vi "CheckForValidPath.vi"(0 "Input VI Path":path, 11 "Error In":errorcluster) -> (4 "Front Panel Reference":refnum<vi>, 6 "VI Reference Out":refnum<vi>, 15 "Error Out":errorcluster)   [LabVIEW 2019, in "JsonToCluster.lvlib"]
doc: "This VI returns the front panel reference of a specified VI if the provided path is valid. If the path is invalid or the VI doesn't exist, it creates a new VI and returns its front panel reference."
uses:
  JsonToCluster.lvlib
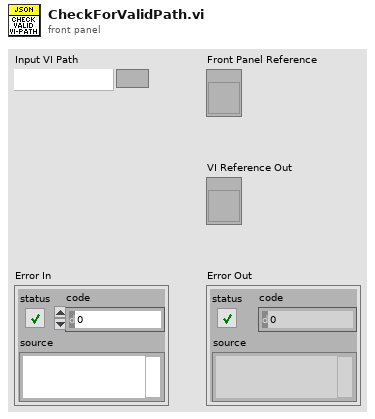
[diagram p1: front panel]
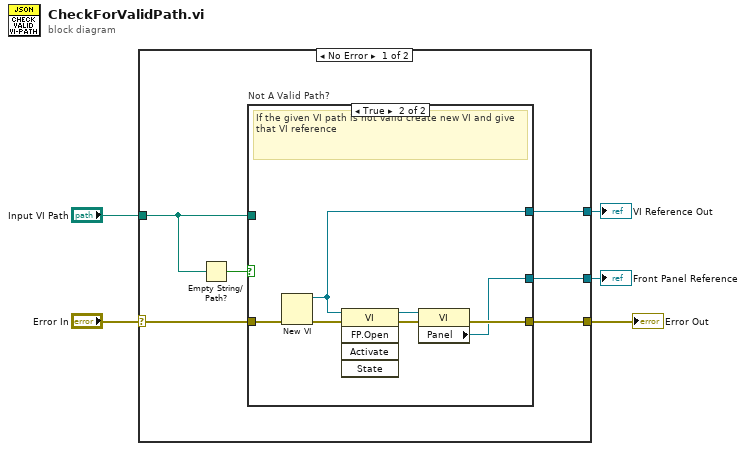
[diagram p0: block diagram]
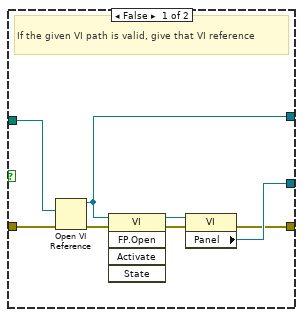
[diagram p2: hidden frame]
diagram:
  n1 = case shown="No Error" "Error In" {
    selector: "Error In" -> [w11 w27]
    tunnel: "Input VI Path" -> [w8 _]
    tunnel: [w10 w27] -> w3
    tunnel: [w9 _] -> w2
    tunnel: [w6 _] -> w1
    frame No Error {
      n2 = Empty String/Path?(string/path=w8) -> (empty?=w7:bool)
      n3 = case "Not A Valid Path?" shown="True" w7 {
        tunnel: w11 -> [w19 w26]
        tunnel: w8 -> [w18 _]
        tunnel: [w14 w21] -> w9
        tunnel: [w13 w22] -> w10
        tunnel: [w12 w20] -> w6
        frame False {
          # "If the given VI path is valid, give that VI reference"
          n4 = Open VI Reference(vi path=w18, error in (no error)=w19) -> (vi reference=w12:refnum<vi>, error out=w15:errorcluster)  [unwired: 4 in]
          n5 = invoke class="VI" method="FP.Open"(reference=w12, error in=w15) -> (reference out=w16:refnum<vi>, error out=w17:errorcluster)  [unwired: 3 in, 3 out]
          n6 = property class="VI"(reference=w16, error in=w17) -> (error out=w13:errorcluster, "Panel"=w14:refnum<vi>)  [unwired: 1 out]
        }
        frame True {
          # "If the given VI path is not valid create new VI and give that VI reference"
          n7 = New VI(8:w26) -> (0:w25:errorcluster, 3:w20:refnum<vi>)  [unwired: 6 in]
          n8 = invoke class="VI" method="FP.Open"(reference=w20, error in=w25) -> (reference out=w23:refnum<vi>, error out=w24:errorcluster)  [unwired: 3 in, 3 out]
          n9 = property class="VI"(reference=w23, error in=w24) -> (error out=w22:errorcluster, "Panel"=w21:refnum<vi>)  [unwired: 1 out]
        }
      }
    }
    frame Error {
    }
  }
  "Error Out" <- w3
  "Front Panel Reference" <- w2
  "VI Reference Out" <- w1
